vi "Page_Advanced_ReadAll.vi"(6 "ctl references":T1, 8 "error in (no error)":errorcluster, 10 "Calculated IncludeHWConfig":bool, 11 "AB_EXE in":refnum<class "AB_EXE.lvclass">) -> (0 "error out":errorcluster, 3 "AB_EXE out":refnum<class "AB_EXE.lvclass">)   [LabVIEW 2020, in "AB_EXE.lvclass"]
uses:
  <vilib>/AppBuilder/AB_Classes/EXE/AB_EXE.lvclass
  e:/builds/penguin/labview/branches/2020/dev/dist/vi.lib/AppBuilder/AB_Classes/TargetFile/AB_Targetfile.lvclass
  <resource>/Framework/Providers/Builds/AppBuilder/AB_UI_Page_Advanced_References.ctl
  <vilib>/AppBuilder/AB_Classes/EXE/AB_EXE.lvclass/AB_EXE.ctl
  <vilib>/AppBuilder/AB_Classes/Application/AB_Application.lvclass
  <vilib>/AppBuilder/AB_Classes/TargetFile/AB_Targetfile.lvclass
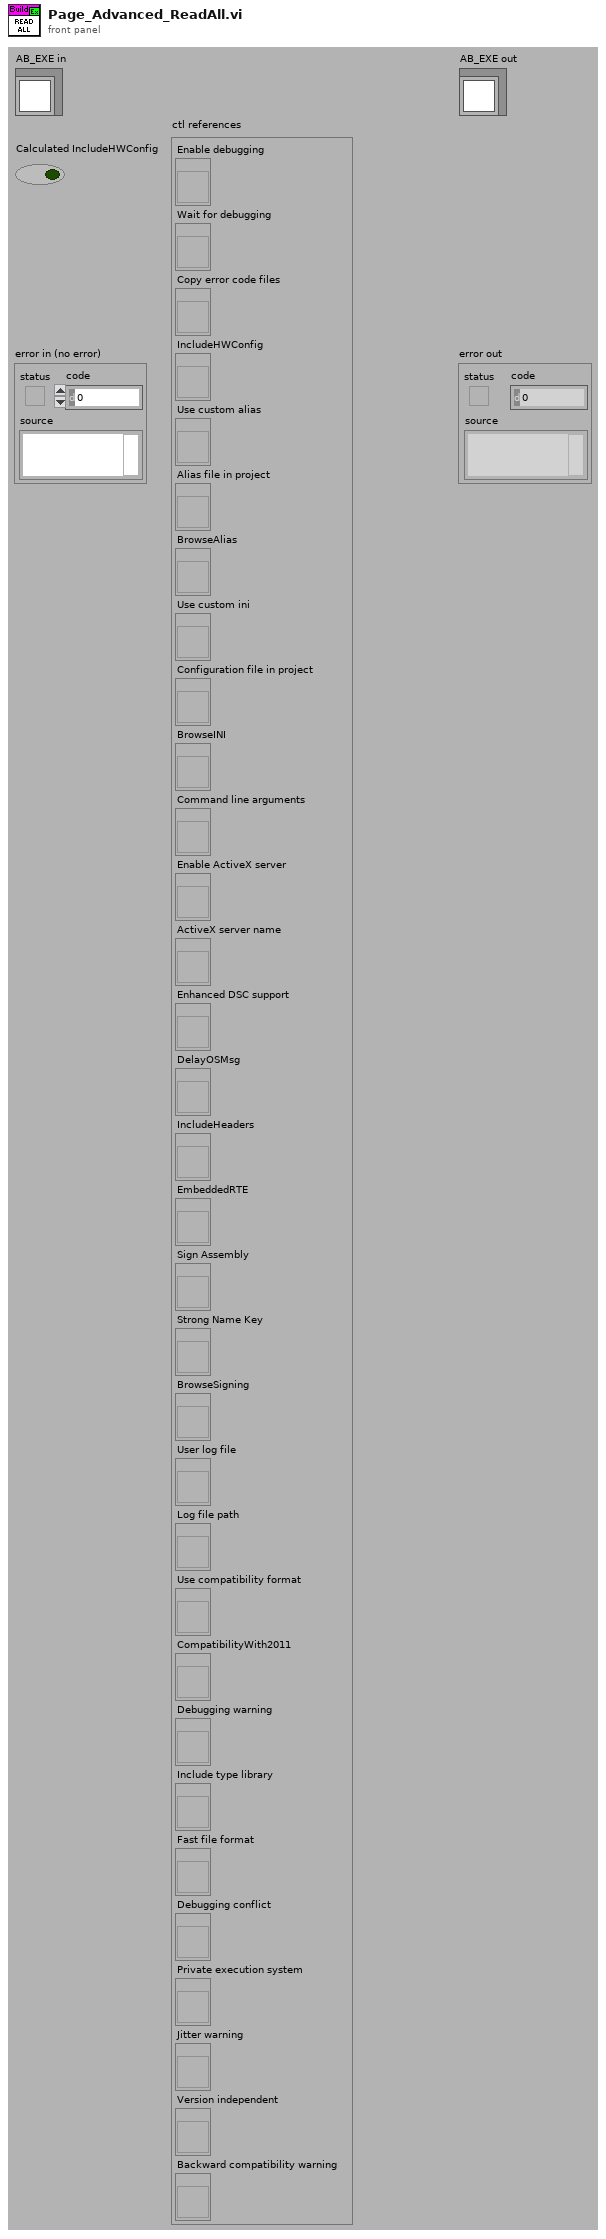
[diagram p1: front panel]
types:
  T1 = typedef "AB_UI_Page_Advanced_References.ctl" = cluster{"Enable debugging":refnum<vi>, "Wait for debugging":refnum<vi>, "Copy error code files":refnum<vi>, "IncludeHWConfig":refnum<vi>, "Use custom alias":refnum<vi>, "Alias file in project":refnum<vi>, "BrowseAlias":refnum<vi>, "Use custom ini":refnum<vi>, "Configuration file in project":refnum<vi>, "BrowseINI":refnum<vi>, "Command line arguments":refnum<vi>, "Enable ActiveX server":refnum<vi>, "ActiveX server name":refnum<vi>, "Enhanced DSC support":refnum<vi>, "DelayOSMsg":refnum<vi>, "IncludeHeaders":refnum<vi>, "EmbeddedRTE":refnum<vi>, "Sign Assembly":refnum<vi>, "Strong Name Key":refnum<vi>, "BrowseSigning":refnum<vi>, "User log file":refnum<vi>, "Log file path":refnum<vi>, "Use compatibility format":refnum<vi>, "CompatibilityWith2011":refnum<vi>, "Debugging warning":refnum<vi>, "Include type library":refnum<vi>, "Fast file format":refnum<vi>, "Debugging conflict":refnum<vi>, "Private execution system":refnum<vi>, "Jitter warning":refnum<vi>, "Version independent":refnum<vi>, "Backward compatibility warning":refnum<vi>}
  T2 = typedef "AB_Targetfile.ctl" = cluster{"targetfileName":string, "targetfileGUID":string, "enableDebugging":bool, "versionInfo":cluster{"productName":string, "legalCopyright":string, "companyName":string, "internalName":string, "fileDescription":string}, "eng_consolidatedTypeInfo":string, "fastFileFormat":bool, "eng_LEIFBuildData":u32, "versionIndependent":bool}
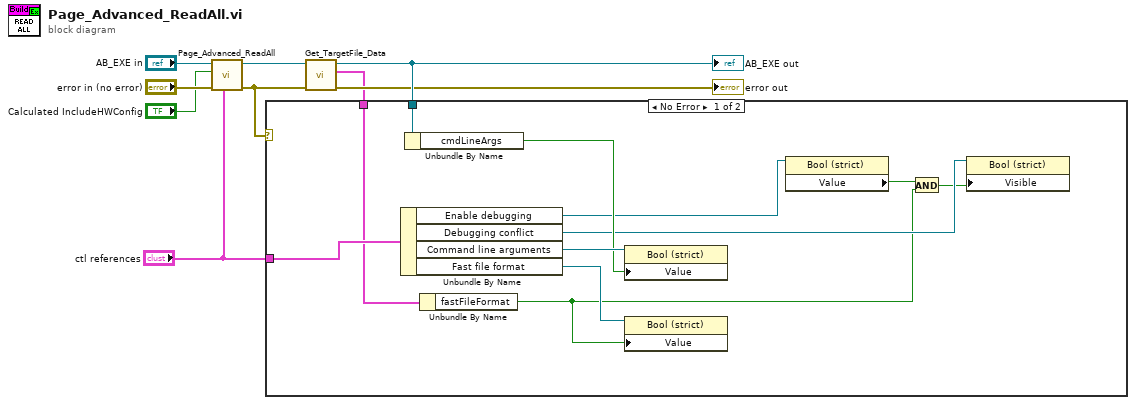
[diagram p0: block diagram]
diagram:
  n1 = call-parent "Page_Advanced_ReadAll.vi"("ctl references"="ctl references", "error in (no error)"="error in (no error)", "Calculated IncludeHWConfig"="Calculated IncludeHWConfig", "AB_Application in"="AB_EXE in") -> ("error out"=w3:errorcluster, "AB_Application out"=w5:refnum<class "AB_EXE.lvclass">)  [unwired: 6 out]
  n2 = call <vilib>:"Get_TargetFile_Data.vi"("error in (no error)"=w3, "AB_Targetfile in"=w5) -> ("error out"=→"error out":errorcluster, "data"=w1:T2, "AB_Targetfile out"=w4:refnum<class "AB_EXE.lvclass">)  [unwired: 7 in]
  "AB_EXE out" <- w4
  n3 = case shown="No Error" w3 {
    tunnel: "ctl references" -> [w20 _]
    tunnel: w4 -> [w19 _]
    tunnel: w1 -> [w16 _]
    frame No Error {
      n4 = Unbundle By Name(w20) -> ("Enable debugging"=w13:refnum<vi>, "Debugging conflict"=w12:refnum<vi>, "Command line arguments"=w18:refnum<vi>, "Fast file format"=w15:refnum<vi>)
      n5 = Unbundle By Name(w19) -> ("cmdLineArgs"=w17:bool)
      n6 = Unbundle By Name(w16) -> ("fastFileFormat"=w10:bool)
      n7 = property class="Bool (strict)"(reference=w18, "Value"=w17) -> ()  [unwired: 1 in, 2 out]
      n8 = property class="Bool (strict)"(reference=w15, "Value"=w10) -> ()  [unwired: 1 in, 2 out]
      n9 = property class="Bool (strict)"(reference=w13) -> ("Value"=w14:bool)  [unwired: 1 in, 2 out]
      n10 = And(x=w14, y=w10) -> (x .and. y?=w11:bool)
      n11 = property class="Bool (strict)"(reference=w12, "Visible"=w11) -> ()  [unwired: 1 in, 2 out]
    }
    frame Error {
    }
  }
